vi "Actor Core.vi"(8 "error in":errorcluster, 11 "Results":refnum<class "Results.lvclass">) -> (0 "error out":errorcluster, 3 "Actor out":refnum<class "Actor.lvclass">)   [LabVIEW 2016, in "Result Actor.lvlib" / "Results.lvclass"]
doc: "This is Actor Core.vi, the main message handling loop for Actors. An actor usually just sits in this loop and processes messages as they arrive. Any error returned by the message Do.vi call will stop the loop, with error code 43 as the cannonical signal to stop with no error sent to caller. Descendants may override that in Handle Error.vi."
uses:
  <userlib>/Common Components/Results/Results.lvclass
  <vilib>/ActorFramework/Stop Msg/Stop Msg.lvclass
  <vilib>/ActorFramework/Actor/Actor.lvclass
  C:/Program Files (x86)/National Instruments/LabVIEW 2016/vi.lib/ActorFramework/Actor/Actor.lvclass
panel:
  out "String":string
  out "Waveform Graph":waveform(dbl)[](graph)
  out "Pass?":bool
  in  "Stop Button":bool
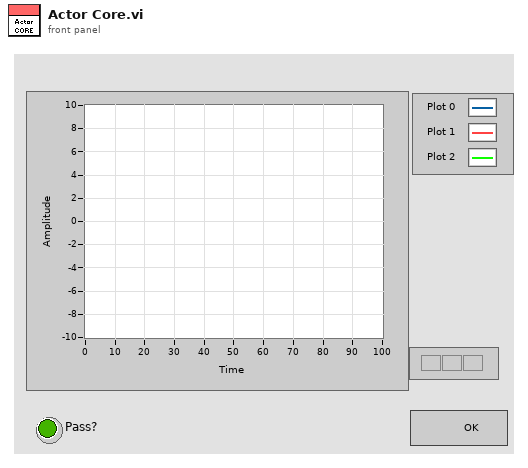
[diagram p1: front panel]
types:
  T1 = cluster{"Stop Button":refnum<vi>, "Waveform Graph":refnum<vi>, "String":refnum<vi>, "Pass?":refnum<vi>}
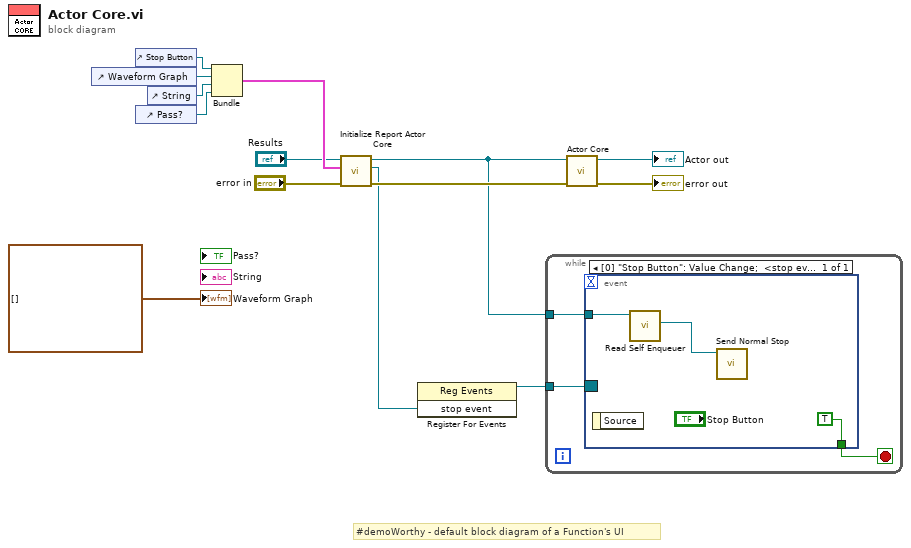
[diagram p0: block diagram]
diagram:
  # "#demoWorthy - default block diagram of a Function's UI"
  n1 = control-ref of="Waveform Graph"() -> (w9:refnum<vi>)
  n2 = control-ref of="Stop Button"() -> (w11:refnum<vi>)
  n3 = control-ref of="Pass?"() -> (w10:refnum<vi>)
  n4 = control-ref of="String"() -> (w12:refnum<vi>)
  n5 = Bundle("Stop Button"=w11, "Waveform Graph"=w9, "String"=w12, "Pass?"=w10) -> (w8:T1)  [unwired: 1 in]
  n6 = call <userlib>:"Initialize Report Actor Core.vi"("error in (no error)"="error in", "Cluster"=w8, "Results in"="Results") -> ("error out"=w5:errorcluster, "stop event"=w1:refnum<user-event>, "Results out"=w4:refnum<class "Results.lvclass">)  [unwired: 6 in]
  n7 = register-events(w1) -> (reference out=w2:refnum<event-registration>)  [unwired: 2 in, 1 out]
  n8 = while {
    tunnel: w4 -> [w16]
    tunnel: w2 -> [w15]
    stop <- w17 stop-if-true
    n9 = event shown="[0] \"Stop Button\": Value Change;  <stop event>: User Event" {
      selector: w15 -> [_]
      dyn-events: _ -> [_]
      timeout: _ -> [_]
      tunnel: [TRUE] -> w17
      tunnel: w16 -> [w19]
      event "Stop Button": Value Change; User Event {
        n10 = event-data() -> ()  [unwired: 1 in, 1 out]
        n11 = call <vilib>:"Read Self Enqueuer.vi"("Actor"=w19) -> ("Self Enqueuer"=w18:refnum<class "Message Enqueuer.lvclass">)  [unwired: 10 in]
        n12 = call <vilib>:"Send Normal Stop.vi"("Message Enqueuer"=w18) -> ()  [unwired: 10 in, 1 out]
      }
    }
  }
  n13 = call-parent "Actor Core.vi"("error in"=w5, "Actor in"=w4) -> ("error out"=→"error out":errorcluster, "Actor out"=→"Actor out":refnum<class "Actor.lvclass">)  [unwired: 8 in]
  "Waveform Graph" <- waveform(dbl)[] [] ("appended array")
